vi "pp3_trial_loadNext.vi"(0 "State Info In":T8={"Curr  tr"=0, "Curr (ms)"=0, "Cum (ms)"=0, "Run loop diff"=0, "Tone countdown (ms)"=0, "Countdown (ms)"=0, "Curr State"=enum."0 NULL", "Prev State"=enum."1 Habituation", "Rw"=FALSE, "Sw"=FALSE, "Tone\nGate"=FALSE, "Punish"=FALSE, "Current DAQ DO Int"=0, "Current Loaded Trial"={"Trial Type Number"=1, "Trial Type"=enum."GO", "Trial Weight"=100, "Shock (mA)"=0.3, "Duration (ms)"=0.25, "Sound Type"=enum."04 FM Sweep", "Stim P1"=4000.0, "Stim P2"=0.0, "Stim P3"=0.0, "Stim P4"=2000.0, "DAQ Amplitude (V)"=0.25}, "Next Trial (for display purposes)"={"Trial Type Number"=1, "Trial Type"=enum."GO", "Trial Weight"=100, "Shock (mA)"=0.3, "Duration (ms)"=0.25, "Sound Type"=enum."04 FM Sweep", "Stim P1"=4000.0, "Stim P2"=0.0, "Stim P3"=0.0, "Stim P4"=2000.0, "DAQ Amplitude (V)"=0.25}, "Total trials memo"=0, "State start cum memo (ms)"=0, "Last dur jump time memo (ms)"=0, "Last dur shock time memo (ms)"=0, "Tone repeat memo (ms)"=0, "Webcam on"=FALSE, "Webcam recording"=FALSE, "State update flag"=FALSE, "Last loaded shock voltage"=0.0, "Vid upd"=enum."0"} {"Current DAQ DO Int" format="%016b"; "Next Trial (for display purposes)"."DAQ Amplitude (V)" min=0.0 max=5.0 format="%_4g"; "Next Trial (for display purposes)"."Shock (mA)" min=-1.0 max=5.0; "Next Trial (for display purposes)"."Trial Weight" step=1; "Next Trial (for display purposes)"."Duration (ms)" min=0.0 max=1.0; "Next Trial (for display purposes)"."Trial Type Number" min=1 max=256 step=1; "Current Loaded Trial"."DAQ Amplitude (V)" min=0.0 max=5.0 format="%_4g"; "Current Loaded Trial"."Shock (mA)" min=-1.0 max=5.0; "Current Loaded Trial"."Trial Weight" step=1; "Current Loaded Trial"."Duration (ms)" min=0.0 max=1.0; "Current Loaded Trial"."Trial Type Number" min=1 max=256 step=1}, 1 "Session param (dynamic)":T7={"Def M shock (uA)"=400.0, "Def F shock (uA)"=0.0}, 2 "Session List (Hidden variable)":u8[](array[numeric]), 3 "Trial Types":T1[](array[typedef])=[{"Trial Type Number"=1, "Trial Type"=enum."GO", "Trial Weight"=1, "Shock (mA)"=-1.0, "Duration (ms)"=250.0, "Sound Type"=enum."04 FM Sweep", "Stim P1"=4000.0, "Stim P2"=0.0, "Stim P3"=0.0, "Stim P4"=2000.0, "DAQ Amplitude (V)"=0.25}, {"Trial Type Number"=2, "Trial Type"=enum."NOGO", "Trial Weight"=1, "Shock (mA)"=-1.0, "Duration (ms)"=250.0, "Sound Type"=enum."04 FM Sweep", "Stim P1"=2000.0, "Stim P2"=0.0, "Stim P3"=0.0, "Stim P4"=4000.0, "DAQ Amplitude (V)"=0.25}] {"DAQ Amplitude (V)" min=0.0 max=5.0 format="%_4g"; "Shock (mA)" min=-1.0 max=5.0; "Trial Weight" step=1; "Duration (ms)" min=0.0 max=1.0; "Trial Type Number" min=1 max=256 step=1}, 5 "Daq config In":T4={"Sound AO"="Dev6/ao0", "Shock intesity AO"="Dev6/ao1", "Code_LED DO"="Dev6/port1:2", "Switch DI"="Dev6/port1/line0", "Webcam"="cam9", "Sound AO task"="", "Sound card task"=0, "Shock intensity AO task"="", "Code_LED DO task"="", "Switch DI task"="", "AO <=> Sound card"=FALSE, "Sound card"=0, "sample rate"=100000.0, "Variable shock"=TRUE, "Webcam on"=FALSE, "Waveform memo"={"t0"=timestamp(0 s since 1904-01-01), "dt"=1.0, "Y"=[]}, "First time"=FALSE, "Tone trigger"="", "Master-9 DO"="Dev6/port0/line5:7", "Master-9 DO task"=""} {"sample rate" min=8000.0; "Sound card task" format="%.0x"}, 7 "log queue in":refnum<queue>, 11 "error in (no error)":errorcluster) -> (4 "State Info Out":T8={"Curr  tr"=0, "Curr (ms)"=0, "Cum (ms)"=0, "Run loop diff"=0, "Tone countdown (ms)"=0, "Countdown (ms)"=0, "Curr State"=enum."0 NULL", "Prev State"=enum."1 Habituation", "Rw"=FALSE, "Sw"=FALSE, "Tone\nGate"=FALSE, "Punish"=FALSE, "Current DAQ DO Int"=0, "Current Loaded Trial"={"Trial Type Number"=1, "Trial Type"=enum."GO", "Trial Weight"=100, "Shock (mA)"=0.3, "Duration (ms)"=0.25, "Sound Type"=enum."04 FM Sweep", "Stim P1"=4000.0, "Stim P2"=0.0, "Stim P3"=0.0, "Stim P4"=2000.0, "DAQ Amplitude (V)"=0.25}, "Next Trial (for display purposes)"={"Trial Type Number"=1, "Trial Type"=enum."GO", "Trial Weight"=100, "Shock (mA)"=0.3, "Duration (ms)"=0.25, "Sound Type"=enum."04 FM Sweep", "Stim P1"=4000.0, "Stim P2"=0.0, "Stim P3"=0.0, "Stim P4"=2000.0, "DAQ Amplitude (V)"=0.25}, "Total trials memo"=0, "State start cum memo (ms)"=0, "Last dur jump time memo (ms)"=0, "Last dur shock time memo (ms)"=0, "Tone repeat memo (ms)"=0, "Webcam on"=FALSE, "Webcam recording"=FALSE, "State update flag"=FALSE, "Last loaded shock voltage"=0.0, "Vid upd"=enum."0"} {"Current DAQ DO Int" format="%016b"; "Next Trial (for display purposes)"."DAQ Amplitude (V)" min=0.0 max=5.0 format="%_4g"; "Next Trial (for display purposes)"."Shock (mA)" min=-1.0 max=5.0; "Next Trial (for display purposes)"."Trial Weight" step=1; "Next Trial (for display purposes)"."Duration (ms)" min=0.0 max=1.0; "Next Trial (for display purposes)"."Trial Type Number" min=1 max=256 step=1; "Current Loaded Trial"."DAQ Amplitude (V)" min=0.0 max=5.0 format="%_4g"; "Current Loaded Trial"."Shock (mA)" min=-1.0 max=5.0; "Current Loaded Trial"."Trial Weight" step=1; "Current Loaded Trial"."Duration (ms)" min=0.0 max=1.0; "Current Loaded Trial"."Trial Type Number" min=1 max=256 step=1}, 8 "log queue out":refnum<queue>, 15 "error out":errorcluster)   [LabVIEW 2013]
doc: "This VI loads the next trial into \"current loaded trial\" in the State info, and applies approrpiate variable shock if applicable"
uses:
  pp3_CTL_StateInfo.ctl
  pp3_CTL_State.ctl
  pp3_CTL_Trial.ctl
  pp3_CTL_TrialType.ctl
  labolabo2/waveforms/WFTypes.ctl
  pp3_CTL_SessionParamDynamic.ctl
  pp3b_CTL_DaqConfig.ctl
  <vilib>/userdefined/High Color/IMAQdx.ctl
  <vilib>/sound2/lvsound2.llb/Sound Output Task ID.ctl
  <vilib>/DAQmx/write.llb/DAQmx Write (Analog 1D DBL 1Chan NSamp).vi
  <vilib>/DAQmx/create/channels.llb/DAQmx Create Channel (AO-Voltage-Basic).vi
  <vilib>/DAQmx/configure/timing.llb/DAQmx Timing (Sample Clock).vi
  <vilib>/DAQmx/miscellaneous.llb/DAQmx Fill In Error Info.vi
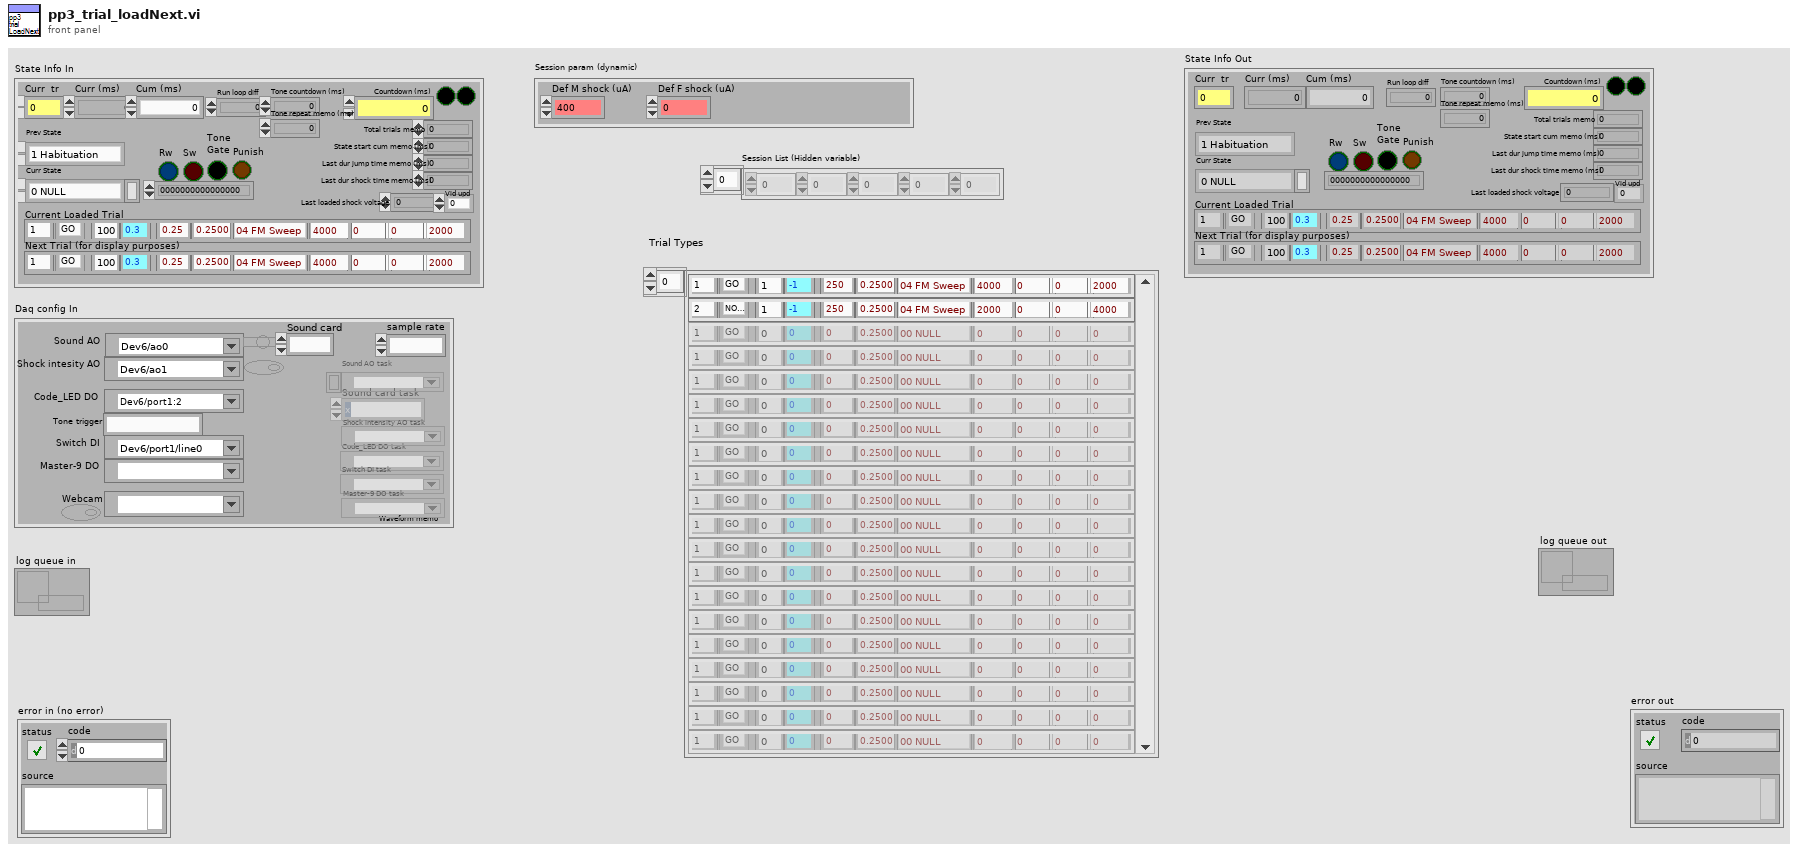
[diagram p1: front panel]
types:
  T1 = typedef "pp3_CTL_Trial.ctl" = cluster{"Trial Type Number":i16, "Trial Type":T2, "Trial Weight":u32, "Shock (mA)":dbl, "Duration (ms)":dbl, "Sound Type":T3, "Stim P1":dbl, "Stim P2":dbl, "Stim P3":dbl, "Stim P4":dbl, "DAQ Amplitude (V)":dbl}
  T2 = typedef "pp3_CTL_TrialType.ctl" = enum16{"OFF", "GO", "NOGO", "TEST"}
  T3 = typedef "WFTypes.ctl" = enum16{"00 NULL", "01 DC", "02 Noise", "03 Pure Tone", "04 FM Sweep"}
  T4 = typedef "pp3b_CTL_DaqConfig.ctl" = cluster{"Sound AO":tag, "Shock intesity AO":tag, "Code_LED DO":tag, "Switch DI":tag, "Webcam":T5, "Sound AO task":refnum<k21>, "Sound card task":T6, "Shock intensity AO task":refnum<k21>, "Code_LED DO task":refnum<k21>, "Switch DI task":refnum<k21>, "AO <=> Sound card":bool, "Sound card":u32, "sample rate":dbl, "Variable shock":bool, "Webcam on":bool, "Waveform memo":waveform(dbl), "First time":bool, "Tone trigger":string, "Master-9 DO":tag, "Master-9 DO task":refnum<k21>}
  T5 = typedef "IMAQdx.ctl" = refnum<k21>
  T6 = typedef "Sound Output Task ID.ctl" = u32
  T7 = typedef "pp3_CTL_SessionParamDynamic.ctl" = cluster{"Def M shock (uA)":dbl, "Def F shock (uA)":dbl}
  T8 = typedef "pp3_CTL_StateInfo.ctl" = cluster{"Curr  tr":u16, "Curr (ms)":u32, "Cum (ms)":i64, "Run loop diff":i64, "Tone countdown (ms)":i64, "Countdown (ms)":i64, "Curr State":T9, "Prev State":T9, "Rw":bool, "Sw":bool, "Tone\nGate":bool, "Punish":bool, "Current DAQ DO Int":u16, "Current Loaded Trial":T1, "Next Trial (for display purposes)":T1, "Total trials memo":i64, "State start cum memo (ms)":i64, "Last dur jump time memo (ms)":i64, "Last dur shock time memo (ms)":i64, "Tone repeat memo (ms)":i64, "Webcam on":bool, "Webcam recording":bool, "State update flag":bool, "Last loaded shock voltage":dbl, "Vid upd":enum16{"0", "1", "2", "3", "4", "5", "6", "7", "8", "9"}}
  T9 = typedef "pp3_CTL_State.ctl" = enum8{"0 NULL", "1 Habituation", "2 (Load Trial)", "3 Stay Period", "4 Load Audio/Click Delay", "5 GO Trial", "6 GO Jumped", "7 GO Timeout", "8 NOGO Trial", "9 NOGO Jumped", "10 NOGO Timeout", "11 TEST Trial", "12 TEST Jumped", "13 TEST Timeout", "14 Intertrial Interval", "15 Done"}
  T10 = typedef "pp2_CTL_DaqConfig.ctl" = cluster{"Sound AO":tag, "Shock intesity AO":tag, "Code_LED DO":tag, "Switch DI":tag, "Webcam":T5, "Sound AO task":refnum<k21>, "Sound card task":T6, "Shock intensity AO task":refnum<k21>, "Code_LED DO task":refnum<k21>, "Switch DI task":refnum<k21>, "AO <=> Sound card":bool, "Sound card":u32, "sample rate":dbl, "Variable shock":bool, "Webcam on":bool, "Tone gate PFI":tag, "Waveform memo":waveform(dbl), "First time":bool}
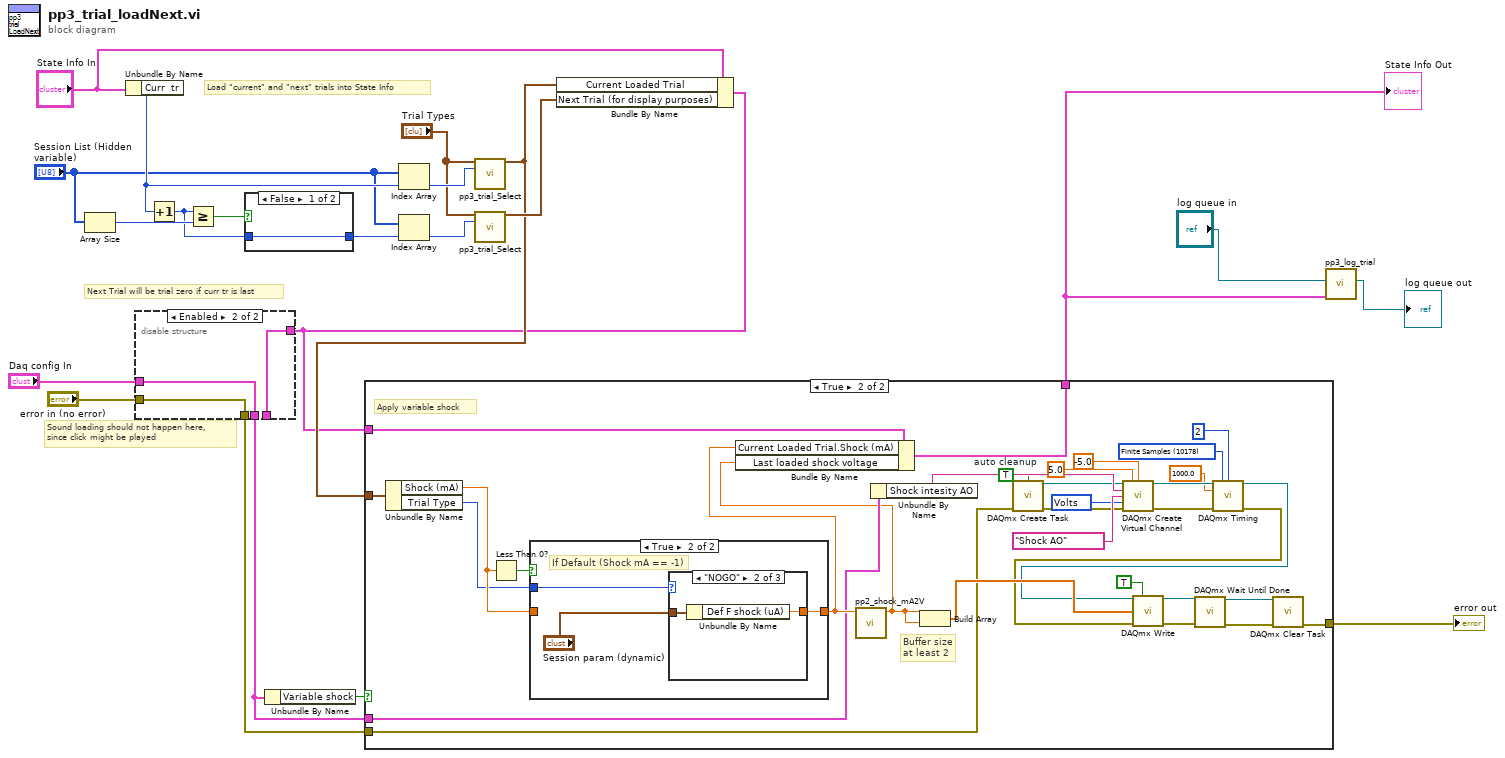
[diagram p0: block diagram]
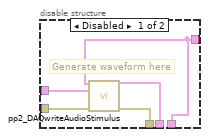
[diagram p2: hidden frame]
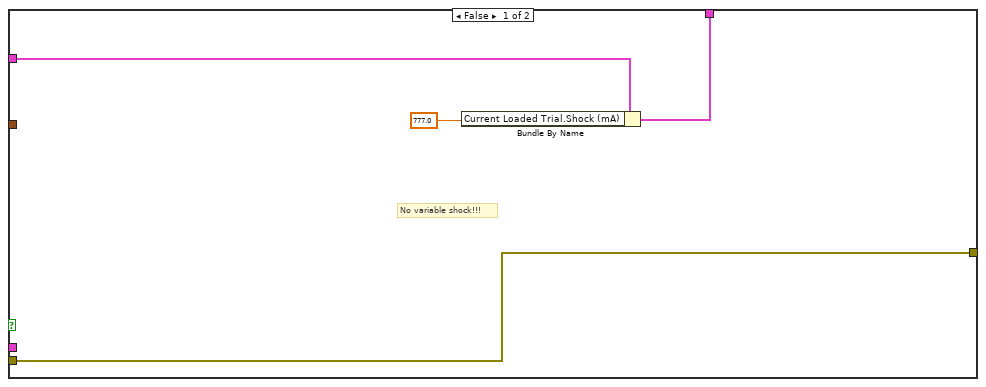
[diagram p3: hidden frame]
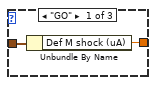
[diagram p5: hidden frame]
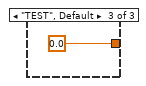
[diagram p6: hidden frame]
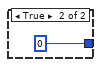
[diagram p7: hidden frame]
diagram:
  # "Load \"current\" and \"next\" trials into State Info"
  # "Sound loading should not happen here,\nsince click might be played"
  # "Next Trial will be trial zero if curr tr is last"
  n1 = Array Size(array="Session List (Hidden variable)") -> (size(s)=w20:i32)
  n2 = Unbundle By Name("State Info In") -> ("Curr  tr"=w18:u16)
  n3 = Increment(x=w18) -> (x+1=w17:u16)
  n4 = Greater Or Equal?(x=w17, y=w20) -> (x >= y?=w19:bool)
  n5 = case shown="False" w19 {
    tunnel: w17 -> [w23 _]
    tunnel: [w23 u8 0] -> w11
    frame False {
    }
    frame True {
    }
  }
  n6 = Index Array(array="Session List (Hidden variable)", index=w18) -> (element=w12:u8)
  n7 = Index Array(array="Session List (Hidden variable)", index=w11) -> (element=w8:u8)
  n8 = call "pp3_trial_Select.vi"("Trial Types"="Trial Types", "Code"=w12) -> ("Cluster 2"=w5:T1)  [unwired: 13 in]
  n9 = call "pp3_trial_Select.vi"("Trial Types"="Trial Types", "Code"=w8) -> ("Cluster 2"=w7:T1)  [unwired: 13 in]
  n10 = Bundle By Name(cluster="State Info In", "Current Loaded Trial"=w5, "Next Trial (for display purposes)"=w7) -> (w4:T8)
  n11 = disable-structure shown="Enabled" {
    disable-tunnel: "Daq config In" -> [w29 w32]
    disable-tunnel: "error in (no error)" -> [w28 w30]
    disable-tunnel: w4 -> [w25 w31]
    disable-tunnel: [w27 w32] -> w6
    disable-tunnel: [w26 w30] -> w13
    disable-tunnel: [w25 w31] -> _
    frame Disabled {
      # "Generate waveform here"
      n12 = call "pp2_DAQwriteAudioStimulus.vi"("State Info In"=w25, "Daq config In"=w29, "error in (no error)"=w28) -> ("Daq config Out"=w27:T10, "error out"=w26:errorcluster)  [unwired: 11 in]
    }
    frame Enabled {
    }
  }
  n13 = Unbundle By Name(w6) -> ("Variable shock"=w21:bool)
  n14 = case shown="True" w21 {
    tunnel: w6 -> [_ w50]
    tunnel: w13 -> [w36 w39]
    tunnel: [w36 w47] -> w16
    tunnel: w4 -> [w34 w65]
    tunnel: [w35 w64] -> w1
    tunnel: w5 -> [_ w63]
    frame False {
      # "No variable shock!!!"
      n15 = Bundle By Name(cluster=w34, "Current Loaded Trial.Shock (mA)"=777.0) -> (w35:T8)
    }
    frame True {
      w40 = TRUE  # auto cleanup
      w53 = 10178 items=["Finite Samples"=10178, "Continuous Samples"=10123, "Hardware Timed Single Point"=12522] ("sample mode")
      w57 = 10348 items=["Volts"=10348, "From Custom Scale"=10065] ("units")
      # "Buffer size\nat least 2"
      # "Apply variable shock"
      n16 = Unbundle By Name(w63) -> ("Shock (mA)"=w67:dbl, "Trial Type"=w66:T2)
      n17 = Less Than 0?(x=w67) -> (x < 0?=w68:bool)
      n18 = case shown="True" w68 {
        tunnel: w66 -> [_ w72]
        tunnel: w67 -> [w69 _]
        tunnel: [w69 w70] -> w61
        frame False {
          # "If 0 or positive shock specification..."
        }
        frame True {
          # "If Default (Shock mA == -1)"
          n19 = case shown="\"NOGO\"" w72 {
            tunnel: "Session param (dynamic)" -> [w74 w76 _]
            tunnel: [w73 w75 0.0 ("Shock (mA)")] -> w70
            frame "GO" {
              n20 = Unbundle By Name(w74) -> ("Def M shock (uA)"=w73:dbl)
            }
            frame "NOGO" {
              n21 = Unbundle By Name(w76) -> ("Def F shock (uA)"=w75:dbl)
            }
            frame "TEST", Default {
            }
          }
        }
      }
      n22 = call "pp2_shock_mA2V.vi"("Shock (mA)"=w61) -> ("Shock (V)"=w44:dbl)  [unwired: 10 in]
      n23 = Bundle By Name(cluster=w65, "Current Loaded Trial.Shock (mA)"=w61, "Last loaded shock voltage"=w44) -> (w64:T8)
      n24 = Unbundle By Name(w50) -> ("Shock intesity AO"=w52:tag)
      n25 = Build Array(w44, w44) -> (w60:dbl[])
      n26 = call <vilib>:"DAQmx Create Task.vi"("auto cleanup"=w40, "error in"=w39) -> ("task out"=w38:refnum<k21>, "error out"=w37:errorcluster)  [unwired: 12 in]
      n27 = call-poly <vilib>:"DAQmx Create Virtual Channel.vi"("task in"=w38, "maximum value"=5.0, "minimum value"=-5.0, "physical channels"=w52, "name to assign"="Shock AO", "units"=w57, "error in"=w37) -> ("task out"=w55:refnum<k21>, "error out"=w54:errorcluster)  [unwired: 7 in]
      n28 = call-poly <vilib>:"DAQmx Timing.vi"("task/channels in"=w55, "sample mode"=w53, "samples per channel"=2, "rate"=1000.0, "error in"=w54) -> ("task out"=w46:refnum<k21>, "error out"=w45:errorcluster)  [unwired: 9 in]
      n29 = call-poly <vilib>:"DAQmx Write.vi"("task/channels in"=w46, "auto start"=TRUE, "data"=w60, "error in"=w45) -> ("task out"=w49:refnum<k21>, "error out"=w48:errorcluster)  [unwired: 9 in, 1 out]
      n30 = call <vilib>:"DAQmx Wait Until Done.vi"("task/channels in"=w49, "error in"=w48) -> ("task out"=w42:refnum<k21>, "error out"=w41:errorcluster)  [unwired: 12 in]
      n31 = call <vilib>:"DAQmx Clear Task.vi"("task in"=w42, "error in"=w41) -> ("error out"=w47:errorcluster)  [unwired: 13 in]
    }
  }
  "State Info Out" <- w1
  "error out" <- w16
  n32 = call "pp3_log_trial.vi"("State Info In"=w1, "queue in"="log queue in") -> ("queue out"=→"log queue out":refnum<queue>)  [unwired: 9 in]
